vi "GenerateSystemDefinitionReport.vi"(8 "error in (no error)":errorcluster, 11 "System Definition Information in":T1) -> (0 "error out":errorcluster, 3 "Target Information String":string)   [LabVIEW 2015, in "VeriStandTestUtilities.lvlib"]
uses:
  VeriStandTestUtilities.lvlib
  SystemDefinitionInformation.ctl
  TargetInformation.ctl
  ChassisInformation.ctl
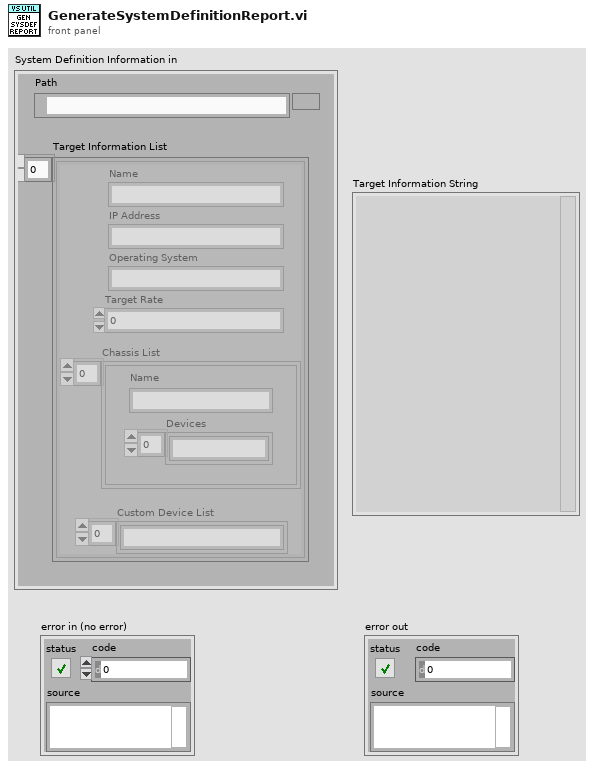
[diagram p1: front panel]
types:
  T1 = typedef "VeriStandTestUtilities.lvlib/SystemDefinitionInformation.ctl" = cluster{"Path":path, "Target Information List":T2[]}
  T2 = typedef "VeriStandTestUtilities.lvlib/TargetInformation.ctl" = cluster{"Name":string, "IP Address":string, "Operating System":string, "Target Rate":dbl, "Chassis List":T3[], "Custom Device List":string[]}
  T3 = typedef "VeriStandTestUtilities.lvlib/ChassisInformation.ctl" = cluster{"Name":string, "Devices":string[]}
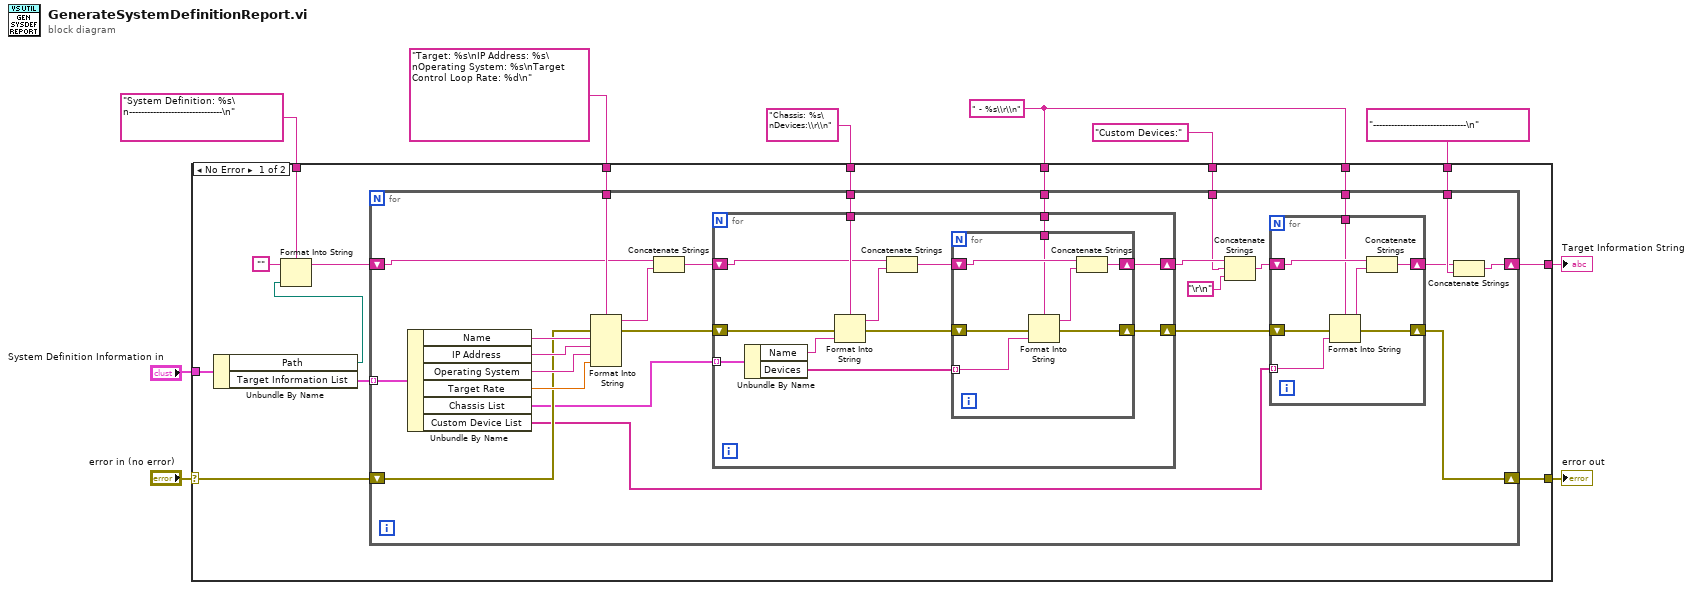
[diagram p0: block diagram]
diagram:
  w3 = " - %s\\r\\n" ("format string")
  n1 = case shown="No Error" "error in (no error)" {
    selector: "error in (no error)" -> [w23 w77]
    tunnel: [w21 w77] -> w9
    tunnel: "System Definition Information in" -> [w25 _]
    tunnel: "Target: %s\nIP Address: %s\nOperating System: %s\nTarget Control Loop Rate: %d\n" ("format string") -> [w24 _]
    tunnel: "Chassis: %s\nDevices:\\r\\n" ("format string") -> [w22 _]
    tunnel: [w20 _] -> w6
    tunnel: "-------------------------------\n" -> [w19 _]
    tunnel: "Custom Devices:" ("string") -> [w18 _]
    tunnel: w3 -> [w17 _]
    tunnel: w3 -> [w16 _]
    tunnel: "System Definition: %s\n-------------------------------\n" ("format string") -> [w11 _]
    frame No Error {
      n2 = Unbundle By Name(w25) -> ("Path"=w13:path, "Target Information List"=w15:T2[])
      n3 = Format Into String(format string=w11, initial string="", w13) -> (resulting string=w14:string)  [unwired: 1 in, 1 out]
      n4 = for {
        tunnel: w15 -> [w50] mode=indexing
        tunnel: w24 -> [w49]
        tunnel: w22 -> [w42]
        shift-right: [w28] -> w21
        shift-left: w23 -> [w44]
        shift-right: [w37] -> w20
        shift-left: w14 -> [w38]
        tunnel: w19 -> [w36]
        tunnel: w18 -> [w31]
        tunnel: w17 -> [w27]
        tunnel: w16 -> [w26]
        n5 = Unbundle By Name(w50) -> ("Name"=w48:string, "IP Address"=w47:string, "Operating System"=w46:string, "Target Rate"=w45:dbl, "Chassis List"=w43:T3[], "Custom Device List"=w35:string[])
        n6 = Format Into String(format string=w49, error in=w44, w48, w47, w46, w45) -> (resulting string=w40:string, error out=w41:errorcluster)  [unwired: 1 in]
        n7 = Concatenate Strings(w38, w40) -> (w39:string)
        n8 = for {
          tunnel: w43 -> [w69] mode=indexing
          tunnel: w42 -> [w68]
          shift-right: [w64] -> w32
          shift-left: w41 -> [w66]
          shift-right: [w60] -> w33
          shift-left: w39 -> [w62]
          tunnel: w27 -> [w58]
          n9 = Unbundle By Name(w69) -> ("Name"=w67:string, "Devices"=w59:string[])
          n10 = Format Into String(format string=w68, error in=w66, w67) -> (resulting string=w63:string, error out=w65:errorcluster)  [unwired: 1 in]
          n11 = Concatenate Strings(w62, w63) -> (w61:string)
          n12 = for {
            tunnel: w59 -> [w76] mode=indexing
            shift-right: [w74] -> w64
            shift-left: w65 -> [w75]
            shift-right: [w73] -> w60
            shift-left: w61 -> [w71]
            tunnel: w58 -> [w70]
            n13 = Format Into String(format string=w70, error in=w75, w76) -> (resulting string=w72:string, error out=w74:errorcluster)  [unwired: 1 in]
            n14 = Concatenate Strings(w71, w72) -> (w73:string)
          }
        }
        n15 = Concatenate Strings(w33, w31, "\r\n") -> (w34:string)
        n16 = for {
          shift-right: [w56] -> w28
          shift-left: w32 -> [w57]
          shift-right: [w52] -> w29
          shift-left: w34 -> [w53]
          tunnel: w35 -> [w55] mode=indexing
          tunnel: w26 -> [w51]
          n17 = Format Into String(format string=w51, error in=w57, w55) -> (resulting string=w54:string, error out=w56:errorcluster)  [unwired: 1 in]
          n18 = Concatenate Strings(w53, w54) -> (w52:string)
        }
        n19 = Concatenate Strings(w29, w36) -> (w37:string)
      }
    }
    frame Error {
    }
  }
  "error out" <- w9
  "Target Information String" <- w6
